vi "Create Fake Detectors.vi"(8 "error in (no error)":errorcluster, 11 "Controller in":refnum<class "Controller.lvclass">) -> (0 "error out":errorcluster, 3 "Controller out":refnum<class "Controller.lvclass">)   [LabVIEW 2019, in "Controller.lvlib" / "Controller.lvclass"]
uses:
  Controller.lvclass
  C:/Program Files (x86)/National Instruments/LabVIEW 2019/vi.lib/ActorFramework/Actor/Actor.lvclass
  Detector Actor/Detector Actor/Detector Actor.lvclass
  Detector Actor/Detector Actor/Detector Actor.lvclass/Detector Actor.ctl
  Sensors/Simulated/Simulated Detector.lvclass
  C:/LabVIEW Sources/MuonDetector/Sensors/Detector/Muon Detector.lvclass
  <vilib>/ActorFramework/Actor/Actor.lvclass
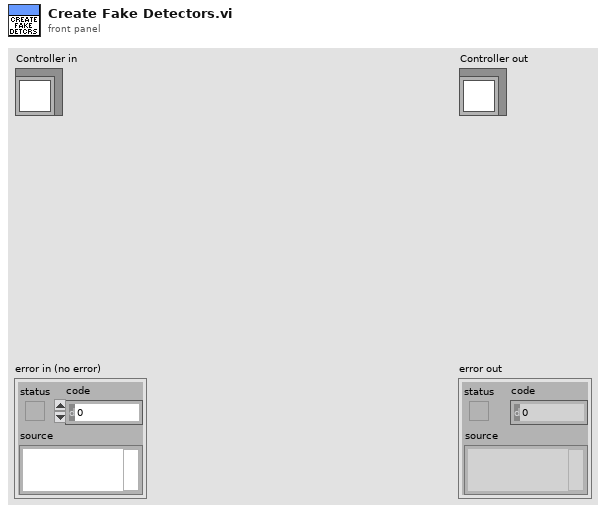
[diagram p1: front panel]
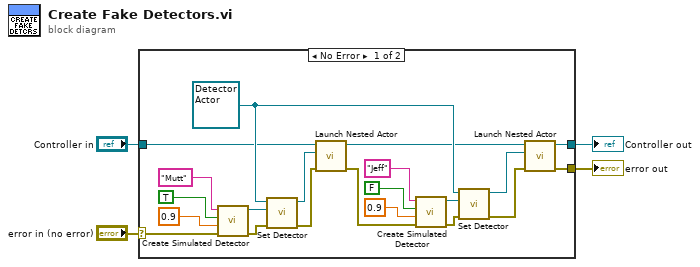
[diagram p0: block diagram]
diagram:
  n1 = case shown="No Error" "error in (no error)" {
    selector: "error in (no error)" -> [w7 w27]
    tunnel: [w9 w27] -> w3
    tunnel: [w11 w26] -> w1
    tunnel: "Controller in" -> [w10 w26]
    frame No Error {
      w23 = refnum<class "Detector Actor.lvclass"> refnum ("Detector Actor.lvlib:Detector Actor.lvclass")
      n2 = call "Create Simulated Detector.vi"("error in (no error)"=w7, "Event Threshold (0-1)"=0.9, "Master"=TRUE, "Name"="Mutt") -> ("error out"=w22:errorcluster, "Simulated Detector out"=w25:refnum<class "Simulated Detector.lvclass">)  [unwired: 6 in]
      n3 = call "Set Detector.vi"("error in (no error)"=w22, "Muon Detector"=w25, "Detector Actor in"=w23) -> ("error out"=w8:errorcluster, "Detector Actor out"=w14:refnum<class "Detector Actor.lvclass">)  [unwired: 7 in]
      n4 = call <vilib>:"Launch Nested Actor.vi"("error in (no error)"=w8, "Nested Actor"=w14, "Caller Actor in"=w10) -> ("error out"=w6:errorcluster, "Caller Actor out"=w12:refnum<class "Controller.lvclass">)  [unwired: 6 in, 1 out]
      n5 = call "Create Simulated Detector.vi"("error in (no error)"=w6, "Event Threshold (0-1)"=0.9, "Master"=FALSE, "Name"="Jeff") -> ("error out"=w21:errorcluster, "Simulated Detector out"=w24:refnum<class "Simulated Detector.lvclass">)  [unwired: 6 in]
      n6 = call "Set Detector.vi"("error in (no error)"=w21, "Muon Detector"=w24, "Detector Actor in"=w23) -> ("error out"=w5:errorcluster, "Detector Actor out"=w13:refnum<class "Detector Actor.lvclass">)  [unwired: 7 in]
      n7 = call <vilib>:"Launch Nested Actor.vi"("error in (no error)"=w5, "Nested Actor"=w13, "Caller Actor in"=w12) -> ("error out"=w9:errorcluster, "Caller Actor out"=w11:refnum<class "Controller.lvclass">)  [unwired: 6 in, 1 out]
    }
    frame Error {
    }
  }
  "error out" <- w3
  "Controller out" <- w1
